vi "save_to_tdms.vi"(5 "data":waveform(dbl)[](array[waveform]), 6 "Hardware params":refnum<vi>[](array[refnum]), 7 "file path":path, 8 "Digitimer params":refnum<vi>[](array[refnum]), 9 "Trial params":refnum<vi>[](array[refnum]), 10 "Trial Count":u16, 11 "Group name":string) -> ()   [LabVIEW 2020]
panel:
  in  "channel name(s) in (Untitled)":string[](array[string])=["torque", "trigger"]
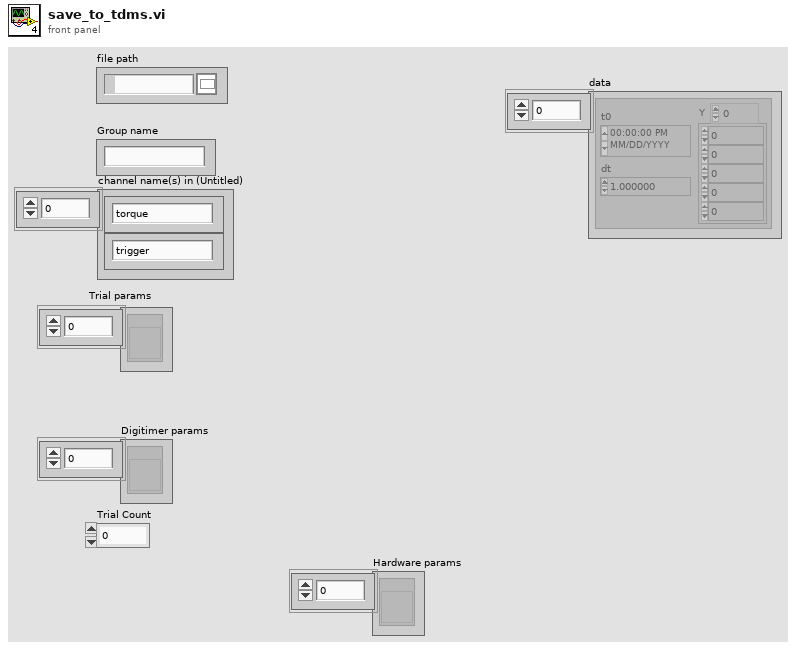
[diagram p1: front panel]
types:
  T1 = enum16{"open", "open or create", "create or replace", "create", "open (read-only)"}
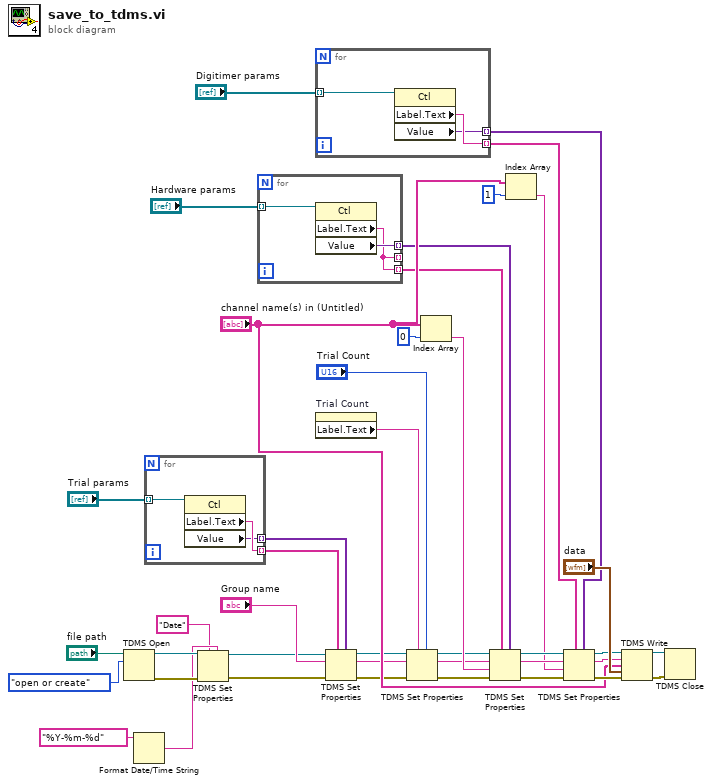
[diagram p0: block diagram]
diagram:
  n1 = TDMS Open(10:T1."open or create" ("operation (0:open)"), 11:"file path") -> (0:w4:errorcluster, 3:w7:refnum<k34>)  [unwired: 5 in]
  n2 = Format Date/Time String(time format string (%c)="%Y-%m-%d") -> (date/time string=w2:string)  [unwired: 2 in]
  n3 = for {
    tunnel: "Trial params" -> [w43] mode=indexing
    tunnel: [w44] -> w29 mode=indexing
    tunnel: [w42] -> w28 mode=indexing
    n4 = property class="Ctl"(reference=w43) -> ("Label.Text"=w44:string, "Value"=w42:variant)  [unwired: 1 in, 2 out]
  }
  n5 = TDMS Set Properties(5:w2, 7:"Date" ("property names"), 8:w4, 11:w7) -> (0:w5:errorcluster, 3:w6:refnum<k34>)  [unwired: 2 in, 2 out]
  n6 = for {
    tunnel: "Hardware params" -> [w47] mode=indexing
    tunnel: [w45] -> _ mode=indexing
    tunnel: [w46] -> w21 mode=indexing
    tunnel: [w45] -> w20 mode=indexing
    n7 = property class="Ctl"(reference=w47) -> ("Label.Text"=w45:string, "Value"=w46:variant)  [unwired: 1 in, 2 out]
  }
  n8 = for {
    tunnel: "Digitimer params" -> [w50] mode=indexing
    tunnel: [w49] -> w18 mode=indexing
    tunnel: [w48] -> w19 mode=indexing
    n9 = property class="Ctl"(reference=w50) -> ("Label.Text"=w49:string, "Value"=w48:variant)  [unwired: 1 in, 2 out]
  }
  n10 = property on="Trial Count" class="DigNum (strict)"() -> ("Label.Text"=w12:string)  [unwired: 2 in, 2 out]
  n11 = TDMS Set Properties(5:w28, 7:w29, 8:w5, 10:"Group name", 11:w6) -> (0:w14:errorcluster, 2:w11:string, 3:w15:refnum<k34>)  [unwired: 1 in, 1 out]
  n12 = TDMS Set Properties(5:"Trial Count", 7:w12, 8:w14, 10:w11, 11:w15) -> (0:w8:errorcluster, 2:w9:string, 3:w10:refnum<k34>)  [unwired: 1 in, 1 out]
  n13 = Index Array(array="channel name(s) in (Untitled)", index=0) -> (element=w17:string)
  n14 = TDMS Set Properties(5:w21, 7:w20, 8:w8, 9:w17, 10:w9, 11:w10) -> (0:w40:errorcluster, 2:w39:string, 3:w38:refnum<k34>)  [unwired: 1 out]
  n15 = Index Array(array="channel name(s) in (Untitled)", index=1) -> (element=w16:string)
  n16 = TDMS Set Properties(5:w19, 7:w18, 8:w40, 9:w16, 10:w39, 11:w38) -> (0:w26:errorcluster, 2:w25:string, 3:w27:refnum<k34>)  [unwired: 1 out]
  n17 = TDMS Write(0:w27, 5:w25, 7:"channel name(s) in (Untitled)", 9:"data", 11:w26) -> (4:w34:refnum<k34>, 15:w33:errorcluster)  [unwired: 1 in, 2 out]
  n18 = TDMS Close(8:w33, 11:w34) -> ()  [unwired: 2 out]
